vi "SIGLENT_SPD3303X-E__VISA__IDN_v01.vi"() -> ()   [LabVIEW 2020]
uses:
  controls/SCPI_enum.ctl
panel:
  in  "Knob":dbl(knob) scale=0.0..32.0
  out "read buffer":string
  in  "SCPI":T1 items=["*IDN?", "*SAV 1", "*RCL 1", "INSTTrument CH1", "INSTTrument CH2", "INSTrument?", "MEASure:CURRent? CH1", "MEASure:CURRent? CH2", "MEASure:VOLTage? CH1", "MEASure:VOLTage? CH2", "MEASure:POWEr? CH1", "MEASure:POWEr? CH2", "CH1:CURRent?", "CH2:CURRent?", "CH1:VOLTage? ", "CH2:VOLTage? ", "OUTPut CH1,ON", "OUTPut CH1,OFF", "OUTPut CH2,ON", "OUTPut CH2,OFF", "OUTPut CH3,ON", "OUTPut CH3,OFF", "OUTPut:TRACK 0", "OUTPut:TRACK 1", "OUTPut:TRACK 2", "OUTPut:WAVE CH1,ON", "OUTPut:WAVE CH1,OFF", "OUTPut:WAVE CH2,ON", "OUTPut:WAVE CH2,OFF"]
  in  "stop":bool
  out "error out":errorcluster
  in  "VISA resource name":refnum<visa-resource-name>
  in  "RUN":bool
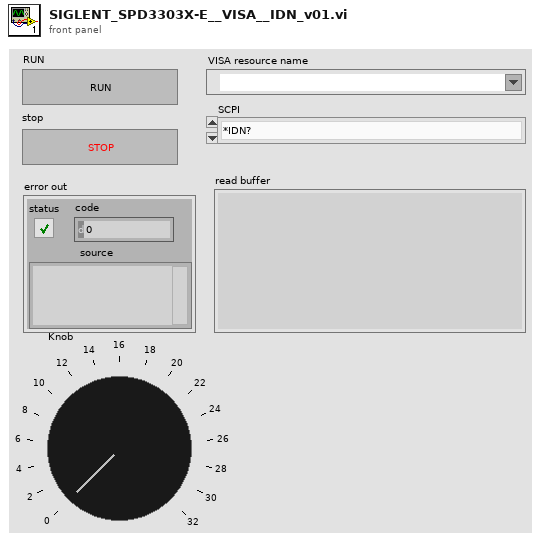
[diagram p1: front panel]
types:
  T1 = typedef "SCPI_enum.ctl" = u16
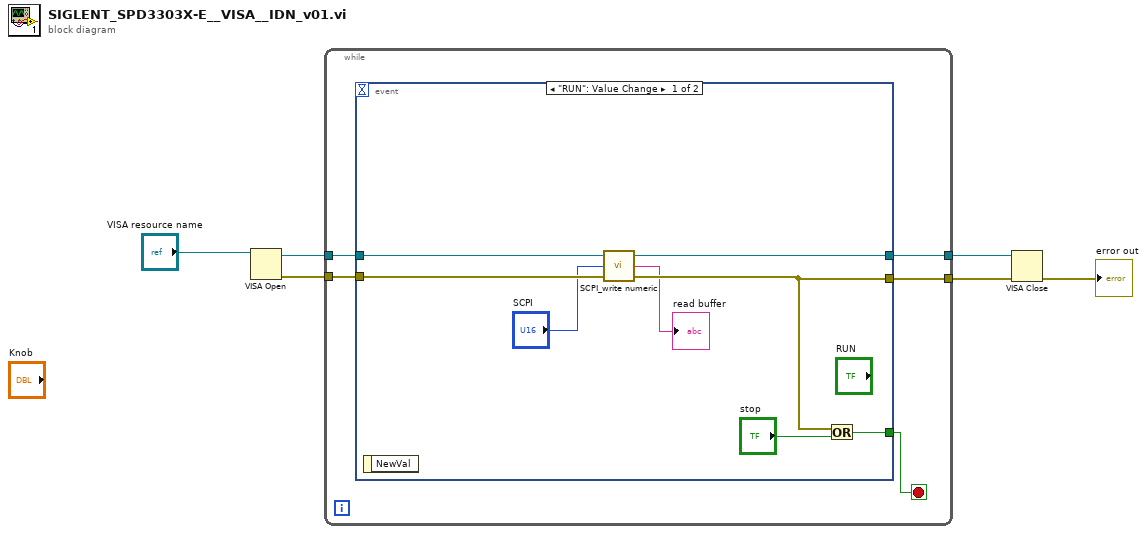
[diagram p0: block diagram]
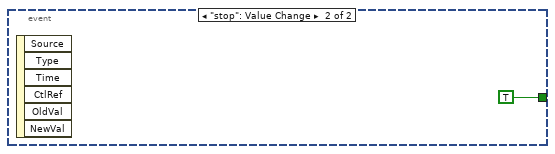
[diagram p2: hidden frame]
diagram:
  n1 = VISA Open(VISA resource name="VISA resource name") -> (VISA resource name=w3:refnum<visa-resource-name>, error out=w4:errorcluster)  [unwired: 4 in]
  n2 = while {
    tunnel: w4 -> [w10]
    tunnel: w3 -> [w9]
    tunnel: [w8] -> w2
    tunnel: [w7] -> w1
    stop <- w11 stop-if-true
    n3 = event shown="[0] \"RUN\": Value Change" {
      selector: _ -> [_ _]
      dyn-events: _ -> [_ _]
      timeout: _ -> [_ _]
      tunnel: [w19 TRUE ("stop")] -> w11
      tunnel: w10 -> [w17 _]
      tunnel: w9 -> [w16 _]
      tunnel: [w14 _] -> w8
      tunnel: [w13 _] -> w7
      event "RUN": Value Change {
        n4 = event-data() -> ()  [unwired: 1 in, 1 out]
        n5 = call "SCPI_write numeric.vi"("error in (no error)"=w17, "SCIPI"="SCPI", "VISA"=w16) -> ("error out"=w14:errorcluster, "read buffer"=→"read buffer":string, "VISA resource name out"=w13:refnum<visa-resource-name>)
        n6 = Or(x=w14, y="stop") -> (x .or. y?=w19:bool)
      }
      event "stop": Value Change {
        n7 = event-data() -> ()  [unwired: 1 in, 6 out]
      }
    }
  }
  n8 = VISA Close(VISA resource name=w1, error in (no error)=w2) -> (error out=→"error out":errorcluster)
